vi "Set NOK in A Row Counter.vi"(8 "error in (no error)":errorcluster, 10 "TestSocketName":string="Counters", 11 "NOK_In_A_Row_Counter":u32) -> (0 "error out":errorcluster)   [LabVIEW 2023, in "Counters.lvlib"]
uses:
  Counters.lvlib
  <vilib>/Utility/config.llb/Write Key (U32).vi
  <vilib>/Utility/config.llb/NI_LVConfig.lvlib
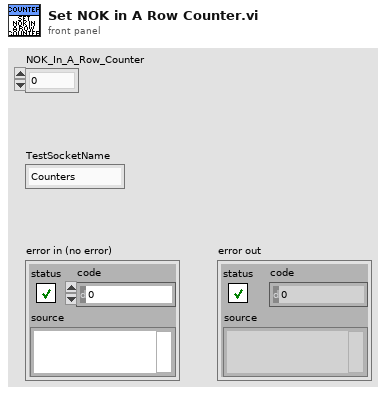
[diagram p1: front panel]
types:
  T1 = typedef "NI_LVConfig.lvlib/Config Data RefNum.ctl" = refnum<k1>
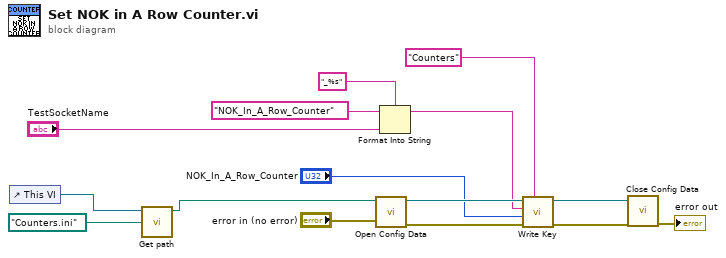
[diagram p0: block diagram]
diagram:
  n1 = control-ref of="This VI"() -> (w6:refnum<vi>)
  n2 = call "Get path.vi"("File mame"=path "Counters.ini" ("configuration file path"), "VI in"=w6) -> ("File path"=w5:path)  [unwired: 9 in]
  n3 = call <vilib>:"Open Config Data.vi"("error in (no error)"="error in (no error)", "configuration file path"=w5) -> ("error out"=w12:errorcluster, "refnum"=w13:T1)  [unwired: 7 in, 1 out]
  n4 = Format Into String(format string="_%s", initial string="NOK_In_A_Row_Counter" ("key"), "TestSocketName") -> (resulting string=w1:string)  [unwired: 1 in, 1 out]
  n5 = call-poly <vilib>:"Write Key.vi"("section"="Counters", "error in (no error)"=w12, "value"="NOK_In_A_Row_Counter", "key"=w1, "refnum"=w13) -> ("error out"=w10:errorcluster, "refnum out"=w11:T1)  [unwired: 4 in, 1 out]
  n6 = call <vilib>:"Close Config Data.vi"("error in (no error)"=w10, "refnum"=w11) -> ("error out"=→"error out":errorcluster)  [unwired: 8 in, 1 out]
